vi "Validate System.vi"(8 "errors in":refnum<class "MultiErrors.lvclass">, 11 "System Config":refnum<class "System Config.lvclass">) -> (0 "errors out":refnum<class "MultiErrors.lvclass">)   [LabVIEW 2020, in "VolatusConfig.lvlib"]
uses:
  VolatusConfig.lvlib
  VolatusErrorUtilities/MultiErrors/MultiErrors.lvclass
  System/System Config.lvclass
  C:/dev/lv20CE/relink/lv-volatus/VolatusConfig/VolatusConfigElement/VolatusConfigElement.lvclass
  VolatusErrorUtilities/MultiErrors/MultiErrors.lvclass/MultiErrors.ctl
  VolatusConfigElement/VolatusConfigElement.lvclass/VolatusConfigElement.ctl
  VolatusConfigElement/Element.vi
  Cluster/Cluster Config.lvclass
  VolatusConfigElement/VolatusConfigElement.lvclass
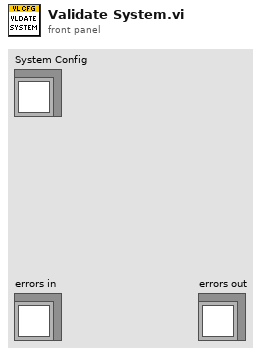
[diagram p1: front panel]
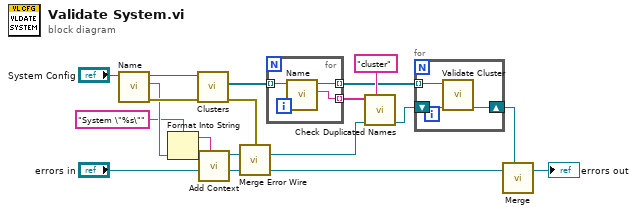
[diagram p0: block diagram]
diagram:
  n1 = call "Name.vi"("VolatusConfigElement in"="System Config") -> ("error out"=w18:errorcluster, "Name"=w14:string, "VolatusConfigElement out"=w15:refnum<class "System Config.lvclass">)  [unwired: 8 in]
  n2 = Format Into String(format string="System \"%s\"" ("Context"), w14) -> (resulting string=w1:string)  [unwired: 2 in, 1 out]
  n3 = call "Clusters.vi"("error in (no error)"=w18, "System Config in"=w15) -> ("error out"=w2:errorcluster, "Clusters"=w9:refnum<class "Cluster Config.lvclass">[])  [unwired: 7 in, 1 out]
  n4 = call "Add Context.vi"("Context"=w1, "MultiErrors in"="errors in") -> ("Original Context"=w12:refnum<class "MultiErrors.lvclass">, "Added Context"=w8:refnum<class "MultiErrors.lvclass">)  [unwired: 8 in]
  n5 = call "Merge Error Wire.vi"("error in (no error)"=w2, "MultiErrors in"=w8) -> ("MultiErrors out"=w3:refnum<class "MultiErrors.lvclass">)  [unwired: 13 in]
  n6 = for {
    tunnel: w9 -> [w21] mode=indexing
    tunnel: [w20] -> w5 mode=indexing
    tunnel: [w19] -> w7 mode=indexing
    n7 = call "Name.vi"("VolatusConfigElement in"=w21) -> ("Name"=w19:string, "VolatusConfigElement out"=w20:refnum<class "Cluster Config.lvclass">)  [unwired: 8 in, 1 out]
  }
  n8 = call "Check Duplicated Names.vi"("Element Type"="cluster", "errors in"=w3, "Names"=w7) -> ("errors out"=w4:refnum<class "MultiErrors.lvclass">)  [unwired: 8 in]
  n9 = for {
    shift-right: [w23] -> w11
    shift-left: w4 -> [w24]
    tunnel: w5 -> [w22] mode=indexing
    n10 = call "Validate Cluster.vi"("errors in"=w24, "Cluster"=w22) -> ("errors out"=w23:refnum<class "MultiErrors.lvclass">)  [unwired: 9 in]
  }
  n11 = call "Merge.vi"("First Error In"=w12, "Second Error In"=w11) -> ("MultiErrors out"=→"errors out":refnum<class "MultiErrors.lvclass">)  [unwired: 5 in]
